vi "Log50mA_Http.vi"(3 "error in (no error)":errorcluster, 5 "LotData in":refnum<class "LotData.lvclass">) -> (0 "error out":errorcluster, 1 "Save Error":bool, 2 "LotData out":refnum<class "LotData.lvclass">)   [LabVIEW 2012, in "LotData.lvclass"]
uses:
  LotData.lvclass
  Controls/JsonTypes/InsertMeasurement.ctl
  Controls/MeasurementType.ctl
  LotData.lvclass/LotData.ctl
  <vilib>/httpClient/PUTBuffer.vi
  <vilib>/LVH/i3 JSON/JSON Parsing/Get Object Parameter Files/Get Object Parameter - Boolean.vi
  <vilib>/LVH/i3 JSON/JSON Parsing/Get Object Parameter Files/Get Object Parameter - String.vi
  <vilib>/httpClient/LabVIEWHTTPClient.lvlib
  <vilib>/LVH/i3 JSON/i3-json.lvlib
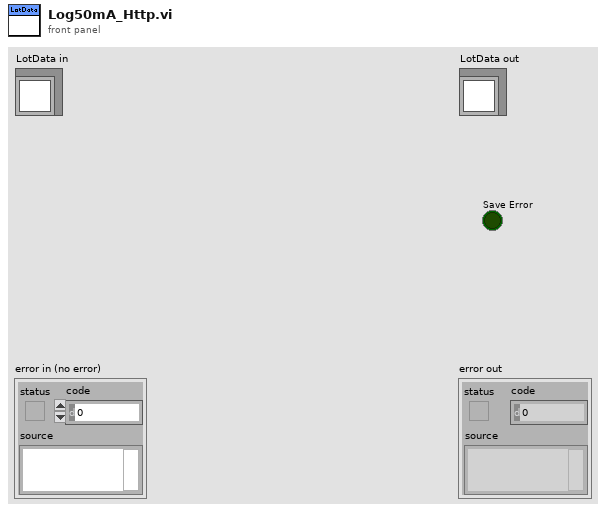
[diagram p1: front panel]
types:
  T1 = typedef "InsertMeasurement.ctl" = cluster{"waferId":string, "actualPad":string, "padLocation":string, "Measurement Type":T2, "Current":dbl, "Power":dbl, "wl":dbl, "voltage":dbl, "knee":dbl, "ir":dbl}
  T2 = typedef "MeasurementType.ctl" = enum16{"Initial", "Final"}
  T3 = typedef "Measurement.ctl" = cluster{"Area":string, "Pad":string, "Current,mA":dbl, "Power":dbl, "WL":dbl, "Voltage":dbl, "Knee Current":dbl, "Reverse":dbl}
  T4 = typedef "LabVIEWHTTPClient.lvlib/ClientHandle.ctl" = refnum<k1>
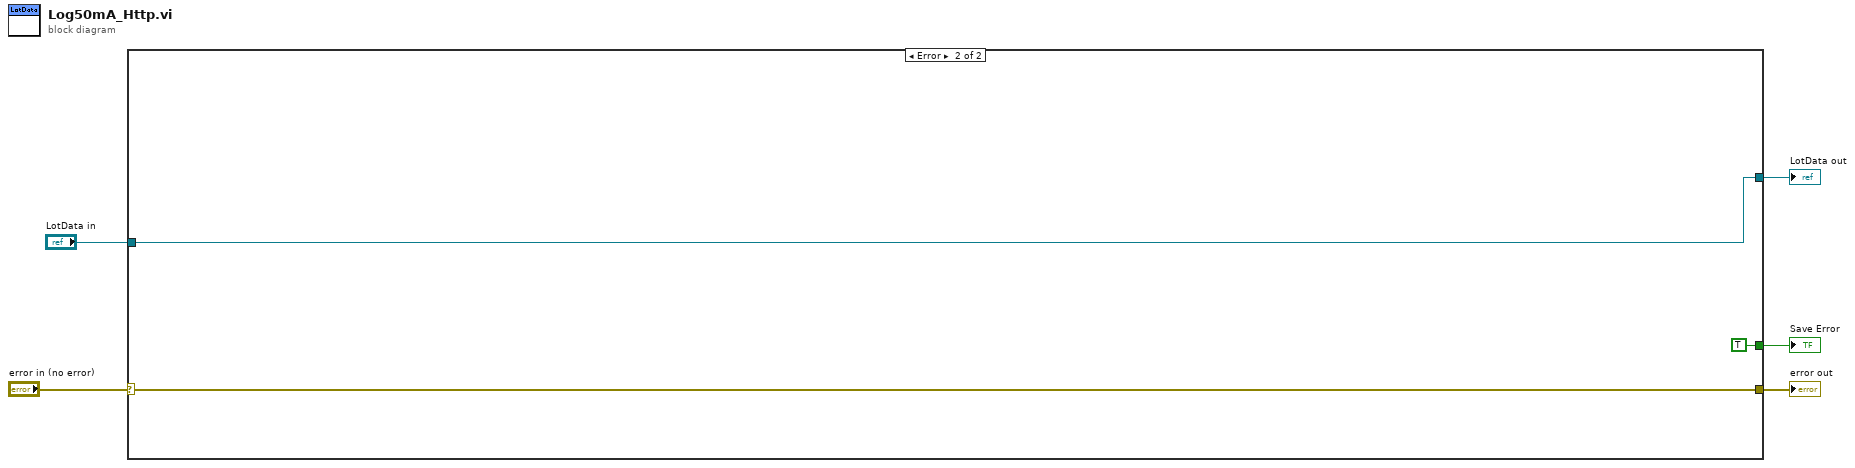
[diagram p0: block diagram]
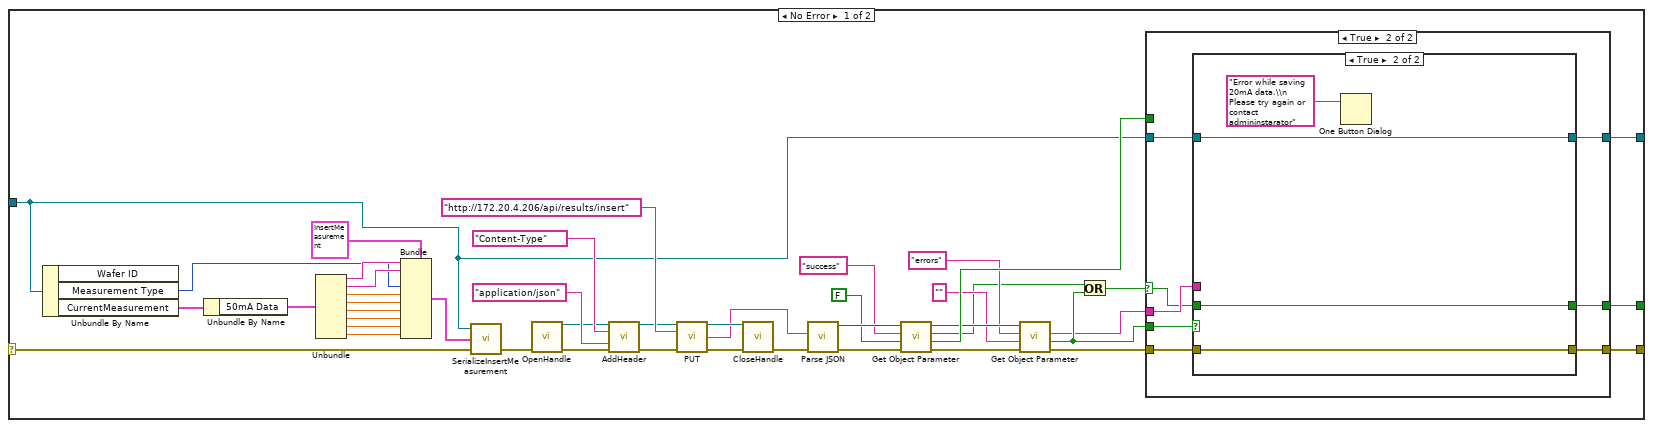
[diagram p2: hidden frame]
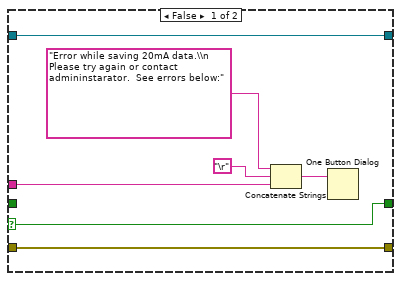
[diagram p4: hidden frame]
diagram:
  n1 = case shown="Error" "error in (no error)" {
    selector: "error in (no error)" -> [w9 w74]
    tunnel: [w8 w74] -> w4
    tunnel: [w6 w73] -> w2
    tunnel: "LotData in" -> [w10 w73]
    tunnel: [w7 TRUE] -> w1
    frame No Error {
      n2 = Unbundle By Name(w10) -> ("Measurement Type"=w38:T2, "CurrentMeasurement"=w49:cluster{"20mA Data":T3, "50mA Data ":T3})  [unwired: 1 out]
      n3 = Unbundle By Name(w49) -> ("50mA Data"=w48:T3)
      n4 = Unbundle(w48) -> ("Area"=w46:string, "Pad"=w45:string, "Current,mA"=w44:dbl, "Power"=w43:dbl, "WL"=w42:dbl, "Voltage"=w39:dbl, "Knee Current"=w41:dbl, "Reverse"=w40:dbl)
      n5 = Bundle(cluster=T1 {"waferId"="", "actualPad"="", "padLocation"="", "Measurement Type"=enum."Initial", "Current"=0.0, "Power"=0.0, "wl"=0.0, "voltage"=0.0, "knee"=0.0, "ir"=0.0} ("InsertMeasurement"), "waferId"=w46, "actualPad"=w45, "Measurement Type"=w38, "Current"=w44, "Power"=w43, "wl"=w42, "voltage"=w39, "knee"=w41, "ir"=w40) -> (w37:T1)  [unwired: 1 in]
      n6 = call-dynamic "SerializeInsertMeasurement.vi"("error in (no error)"=w9, "InsertMeasurement"=w37, "LotData in"=w10) -> ("error out"=w36:errorcluster)  [unwired: 2 out]
      n7 = call <vilib>:"OpenHandle.vi"("error in (no error)"=w36) -> ("client handle out"=w28:T4, "error out"=w27:errorcluster)  [unwired: 13 in]
      n8 = call <vilib>:"AddHeader.vi"("client handle"=w28, "header"="Content-Type", "value"="application/json", "error in (no error)"=w27) -> ("client handle out"=w29:T4, "error out"=w30:errorcluster)  [unwired: 10 in]
      n9 = call-poly <vilib>:"PUT.vi"("client handle"=w29, "url"="http://172.20.4.206/api/results/insert", "error in (no error)"=w30) -> ("client handle out"=w34:T4, "body"=w26:string, "error out"=w33:errorcluster)  [unwired: 9 in, 1 out]
      n10 = call <vilib>:"CloseHandle.vi"("client handle"=w34, "error in (no error)"=w33) -> ("error out"=w25:errorcluster)  [unwired: 13 in]
      n11 = call <vilib>:"Parse JSON.vi"("error in (no error)"=w25, "JSON String"=w26) -> ("error out"=w23:errorcluster, "JSON Tree"=w24:variant)  [unwired: 6 in, 2 out]
      n12 = call-poly <vilib>:"Get Object Parameter.vi"("error in (no error)"=w23, "Default Value if JSON Null"=FALSE, "Parameter Name"="success", "JSON Tree In (JSON Object)"=w24) -> ("error out"=w19:errorcluster, "is JSON Null?"=w21:bool, "Boolean Value"=w14:bool, "JSON Tree Out Passthrough"=w20:variant)  [unwired: 4 in]
      n13 = call-poly <vilib>:"Get Object Parameter.vi"("error in (no error)"=w19, "Default Value if JSON Null"="", "Parameter Name"="errors", "JSON Tree In (JSON Object)"=w20) -> ("error out"=w11:errorcluster, "is JSON Null?"=w15:bool, "String Value"=w13:string)  [unwired: 4 in, 1 out]
      n14 = Or(x=w14, y=w15) -> (x .or. y?=w16:bool)
      n15 = case shown="True" w16 {
        selector: w16 -> [w52 w53]
        tunnel: w21 -> [_ _]
        tunnel: w15 -> [_ w60]
        tunnel: w13 -> [_ w59]
        tunnel: [w52 w54] -> w7
        tunnel: w10 -> [w51 w57]
        tunnel: [w51 w58] -> w6
        tunnel: [w50 w56] -> w8
        tunnel: w11 -> [w50 w55]
        frame False {
        }
        frame True {
          n16 = case shown="True" w60 {
            selector: w60 -> [w61 _]
            tunnel: w59 -> [w65 _]
            tunnel: [w64 w70] -> w58
            tunnel: w57 -> [w64 w70]
            tunnel: [w62 w69] -> w56
            tunnel: w55 -> [w62 w69]
            tunnel: [w61 w68] -> w54
            tunnel: w53 -> [_ w68]
            frame False {
              n17 = Concatenate Strings("Error while saving 20mA data.\\n Please try again or contact admininstarator.  See errors below:" ("message"), "\r", w65) -> (w63:string)
              n18 = One Button Dialog(message=w63) -> ()  [unwired: 1 in, 1 out]
            }
            frame True {
              n19 = One Button Dialog(message="Error while saving 20mA data.\\n Please try again or contact admininstarator") -> ()  [unwired: 1 in, 1 out]
            }
          }
        }
      }
    }
    frame Error {
    }
  }
  "error out" <- w4
  "LotData out" <- w2
  "Save Error" <- w1
